vi "fgv_ekf_process-val.vi"(7 "cmd":T3, 11 "process val":T2) -> (3 "process val out":T2)   [LabVIEW 2019]
uses:
  Ctrl/cmd_common.ctl
  <vilib>/Analysis/Matrix/Datatypes/RealMatrix.ctl
  <vilib>/Analysis/Matrix/NI_Matrix.lvlib
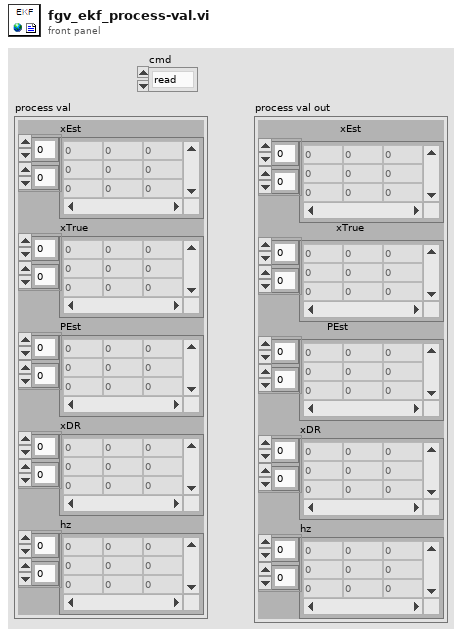
[diagram p1: front panel]
types:
  T1 = typedef "NI_Matrix.lvlib/RealMatrix.ctl" = dbl[][]
  T2 = cluster{"xEst":T1, "xTrue":T1, "PEst":T1, "xDR":T1, "hz":T1}
  T3 = typedef "cmd_common.ctl" = enum16{"read", "write"}
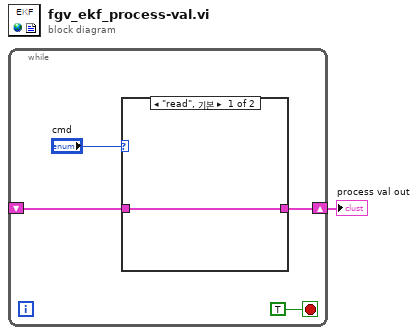
[diagram p0: block diagram]
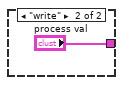
[diagram p2: hidden frame]
diagram:
  n1 = while {
    shift-right: [w3] -> w1
    shift-left: _ -> [w2]
    stop <- TRUE stop-if-true
    n2 = case shown="\"read\", 기본" "cmd" {
      tunnel: [w6 "process val"] -> w3
      tunnel: w2 -> [w6 _]
      frame "read", Default {
      }
      frame "write" {
      }
    }
  }
  "process val out" <- w1
